vi "Error Query.vi"(4 "error in (no error)":errorcluster, 7 "VISA resource name":refnum<visa-resource-name>) -> (0 "error out":errorcluster, 1 "Error Message":string, 2 "Error Code":i32[](array[numeric]), 3 "VISA resource name out":refnum<visa-resource-name>)   [LabVIEW 2010, in "Newport ESP301.lvlib"]
doc: "Queries the instrument for any errors in the instrument's error queue. It will continue to read errors until all errors have been read from the instrument. Any errors will be returned in the <B>error out</B> control."
uses:
  <userlib>/Newport ESP301/Newport ESP301.lvlib
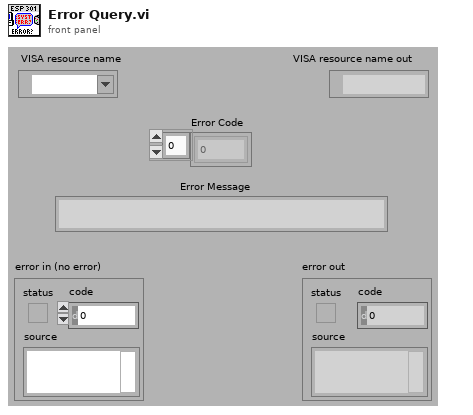
[diagram p1: front panel]
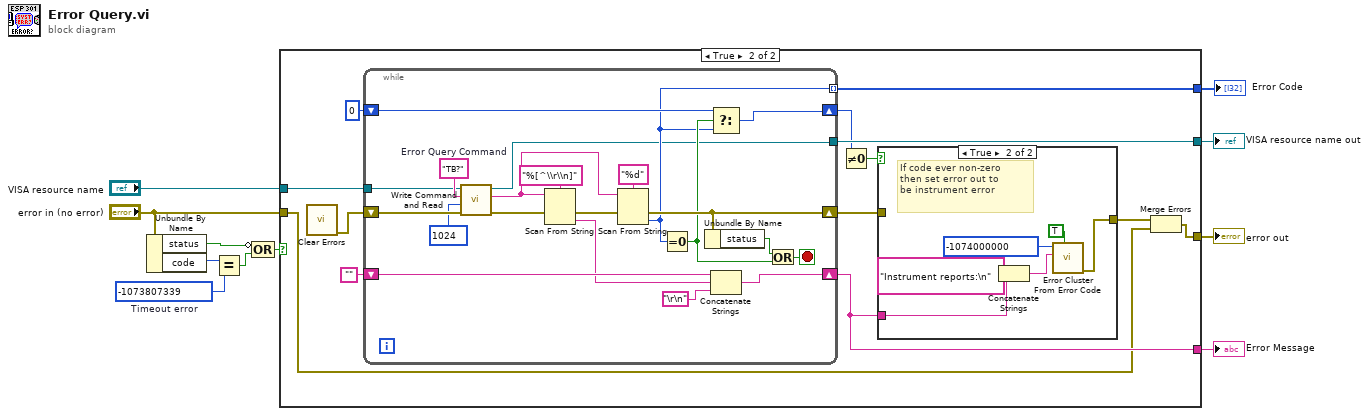
[diagram p0: block diagram]
diagram:
  w6 = -1073807339  # Timeout error
  n1 = Unbundle By Name("error in (no error)") -> ("status"=w7:bool, "code"=w4:i32)
  n2 = Equal?(x=w4, y=w6) -> (x = y?=w5:bool)
  n3 = Compound Arithmetic op=OR(invert w7, w5) -> (w3:bool)
  n4 = case shown="True" w3 {
    tunnel: [w15 w28] -> w11
    tunnel: "VISA resource name" -> [w15 w27]
    tunnel: "error in (no error)" -> [w14 w18]
    tunnel: [w14 w25] -> w9
    tunnel: ["" w20] -> w2
    tunnel: [i32[] [] w19] -> w1
    frame False {
    }
    frame True {
      n5 = call <vilib>:"Clear Errors.vi"() -> ("error out"=w16:errorcluster)  [unwired: 7 in]
      n6 = while {
        tunnel: [w39] -> w28
        tunnel: w27 -> [w40]
        shift-right: [w50] -> w20
        shift-left: "" -> [w53]
        shift-right: [w48] -> w21
        shift-left: 0 -> [w49]
        shift-right: [w47] -> w17
        shift-left: w16 -> [w42]
        tunnel: [w43] -> w19 mode=indexing
        stop <- w55 stop-if-true
        w41 = "TB?"  # Error Query Command
        n7 = call <userlib>:"Write Command and Read.vi"("error in (no error)"=w42, "Bytes to read (100)"=u32 1024, "Command"=w41, "VISA resource name"=w40) -> ("error out"=w38:errorcluster, "Returned string"=w37:string, "VISA resource name out"=w39:refnum<visa-resource-name>)  [unwired: 3 in]
        n8 = Scan From String(format string="%[^\\r\\n]", input string=w37, error in=w38) -> (error out=w46:errorcluster, output 1=w51:string)  [unwired: 2 in, 2 out]
        n9 = Scan From String(format string="%d", input string=w37, error in=w46) -> (error out=w47:errorcluster, output 1=w43:i32)  [unwired: 2 in, 2 out]
        n10 = Equal To 0?(x=w43) -> (x = 0?=w44:bool)
        n11 = Unbundle By Name(w47) -> ("status"=w45:bool)
        n12 = Select(t=w49, s=w44, f=w43) -> (s? t:f=w48:i32)
        n13 = Concatenate Strings(w53, w51, "\r\n") -> (w50:string)
        n14 = Or(x=w45, y=w44) -> (x .or. y?=w55:bool)
      }
      n15 = Not Equal To 0?(x=w21) -> (x != 0?=w23:bool)
      n16 = case shown="True" w23 {
        tunnel: w20 -> [_ w34]
        tunnel: [w29 w30] -> w22
        tunnel: w17 -> [w29 _]
        frame False {
        }
        frame True {
          # "If code ever non-zero\nthen set error out to\nbe instrument error"
          n17 = Concatenate Strings("Instrument reports:\n" ("Source"), w34) -> (w31:string)
          n18 = call <vilib>:"Error Cluster From Error Code.vi"("show call chain? (False)"=TRUE, "error message (\"\")"=w31, "error code (0)"=-1074000000 ("Code")) -> ("error out"=w30:errorcluster)  [unwired: 6 in]
        }
      }
      n19 = Merge Errors(w22, w18) -> (w25:errorcluster)
    }
  }
  "VISA resource name out" <- w11
  "error out" <- w9
  "Error Message" <- w2
  "Error Code" <- w1
